vi "seguidor_parede_odometria.vi"(3 "Text":string, 4 "Line":i16(ring) items=["1", "2", "3", "4", "5", "6", "7", "8", "9", "10", "11", "12"], 5 "NXT/EV3 3":T1) -> (0 "Numeric":dbl format="%#_13g", 2 "NXT/EV3 2":T1)   [LabVIEW 2016]
uses:
  <vilib>/NXT/Subs/LVHSConnector.ctl
  <vilib>/NXT/LegoClasses/BrickReference/BrickReference.lvclass
  <vilib>/NXT/Block Support/NXT_OutputPort.ctl
  <vilib>/NXT/Block Support/NXT_InputPort.ctl
  <vilib>/NXT/Dual Mode Library/Motors/ResetMotor.vi
  <vilib>/NXT/NXTIO Xnodes/NXTIONodeSubVIs/NXTMoveMotors.vi
  <vilib>/NXT/Dual Mode Library/Sensors/EV3_Ultrasonic_CM.vi
  <vilib>/NXT/Dual Mode Library/Sensors/Touch_Pressed.vi
  <vilib>/NXT/Dual Mode Library/Motors/Rotation.vi
  <vilib>/NXT/Dual Mode Library/Display/drawText.vi
  <vilib>/NXT/Dual Mode Library/Display/drawNumber_float.vi
  <vilib>/NXT/NXTIO Xnodes/AddressXNode/NXTIOAddress.xnode
  <vilib>/NXT/NXTIO Xnodes/NXTIOXNode/NXTIO.xnode
panel:
  in  "KE 2":dbl=-0.0356
  in  "Kp":sgl
  in  "Dmin":sgl
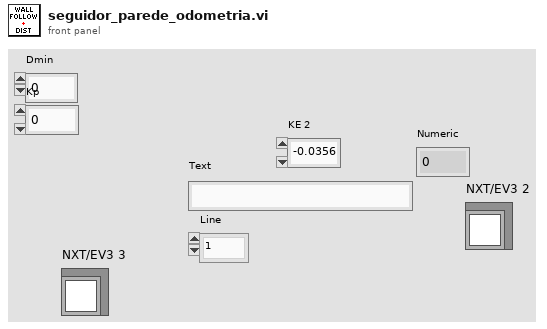
[diagram p1: front panel]
types:
  T1 = typedef "LVHSConnector.ctl" = refnum<class "BrickReference.lvclass">
  T2 = typedef "NXT_OutputPort.ctl" = u8
  T3 = typedef "NXT_InputPort.ctl" = u32
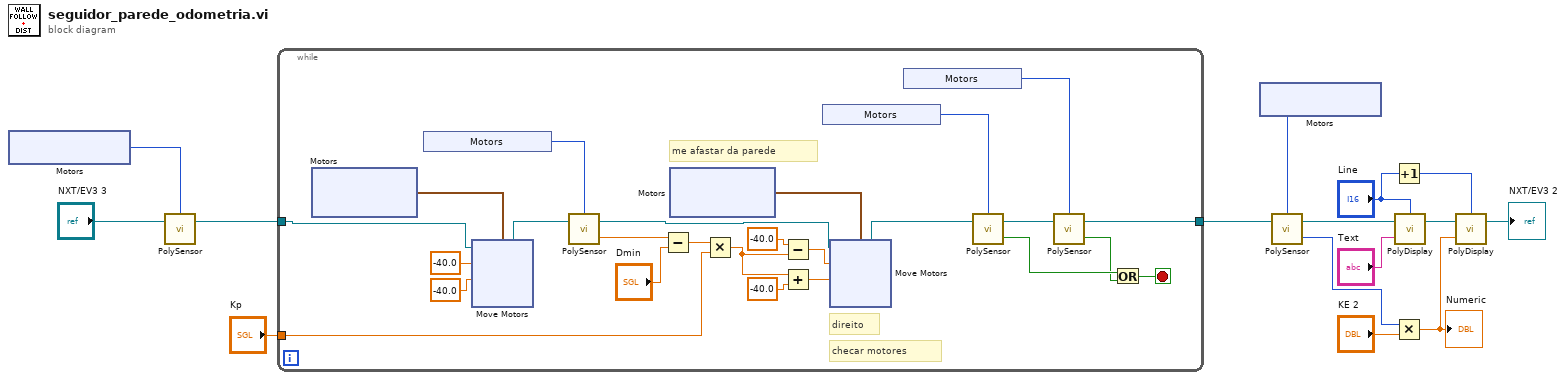
[diagram p0: block diagram]
diagram:
  n1 = xnode "Motors"() -> ("Motor"=w14:T2)
  n2 = call-poly <vilib>:"PolySensor.vi"("NXT/EV3"="NXT/EV3 3", "Port (All Ports)"=w14) -> ("NXT/EV3"=w12:T1)  [unwired: 2 out]
  n3 = while {
    tunnel: w12 -> [w37]
    tunnel: [w25] -> w1
    tunnel: "Kp" -> [w34]
    stop <- w22 stop-if-true
    # "direito"
    # "me afastar da parede"
    # "checar motores"
    n4 = xnode "Motors"() -> ("Motor"=w39:cluster{"Port":T2, "Port":T2})
    n5 = xnode "Motors"() -> ("Sensor"=w21:T3)
    n6 = xnode "Move Motors"("Power/Speed 2"=sgl -40.0 ("x"), "Power/Speed 1"=sgl -40.0 ("x"), "Motors"=w39, "NXT/EV3"=w37) -> ("NXT/EV3"=w38:T1)
    n7 = call-poly <vilib>:"PolySensor.vi"("NXT/EV3"=w38, "Port (Port 1)"=w21) -> ("Centimeters"=w17:sgl, "NXT/EV3"=w40:T1)  [unwired: 1 in]
    n8 = Subtract(x=w17, y="Dmin") -> (x-y=w30:sgl)
    n9 = xnode "Motors"() -> ("Motor"=w31:cluster{"Port":T2, "Port":T2})
    n10 = Multiply(x=w30, y=w34) -> (x*y=w32:sgl)
    n11 = Subtract(x=sgl -40.0, y=w32) -> (x-y=w28:sgl)
    n12 = Add(x=w32, y=sgl -40.0 ("x")) -> (x+y=w29:sgl)
    n13 = xnode "Motors"() -> ("Sensor"=w20:T3)
    n14 = xnode "Move Motors"("Power/Speed 2"=w29, "Power/Speed 1"=w28, "Motors"=w31, "NXT/EV3"=w40) -> ("NXT/EV3"=w26:T1)
    n15 = xnode "Motors"() -> ("Sensor"=w19:T3)
    n16 = call-poly <vilib>:"PolySensor.vi"("NXT/EV3"=w26, "Port (Port 1)"=w20) -> ("Yes / No"=w24:bool, "NXT/EV3"=w27:T1)  [unwired: 1 in]
    n17 = call-poly <vilib>:"PolySensor.vi"("NXT/EV3"=w27, "Port (Port 1)"=w19) -> ("Yes / No"=w23:bool, "NXT/EV3"=w25:T1)  [unwired: 1 in]
    n18 = Or(x=w24, y=w23) -> (x .or. y?=w22:bool)
  }
  n19 = xnode "Motors"() -> ("Motor"=w11:T2)
  n20 = call-poly <vilib>:"PolySensor.vi"("NXT/EV3"=w1, "Port (Port A)"=w11) -> ("Angle of Rotation"=w8:i32, "NXT/EV3"=w7:T1)  [unwired: 1 out]
  n21 = Increment(x="Line") -> (x+1=w3:i16)
  n22 = Multiply(x=w8, y="KE 2") -> (x*y=w2:dbl)
  "Numeric" <- w2
  n23 = call-poly <vilib>:"PolyDisplay.vi"("Text"="Text", "NXT/EV3"=w7, "Line"="Line") -> ("NXT/EV3"=w6:T1)  [unwired: 1 in]
  n24 = call-poly <vilib>:"PolyDisplay.vi"("number"=w2, "NXT/EV3"=w6, "Line"=w3) -> ("NXT/EV3"=→"NXT/EV3 2":T1)  [unwired: 1 in]
